vi "Generate Text Coordenates.vi"(8 "Error In":errorcluster, 11 "Pixel In":refnum<class "String.lvclass">) -> (0 "Error Out":errorcluster, 2 "Element To Display":T1[](array[typedef]), 3 "Pixel Out":refnum<class "String.lvclass">)   [LabVIEW 2019, in "String.lvclass"]
uses:
  String.lvclass
  C:/Users/goo13/Documents/GIT Local/myRIO-Neopixel/Source/RT/Display Element/Display Element.lvclass
  Display Utilities/Public/Controls/2D Coordenates.ctl
  Display Utilities/Display Utilities.lvlib
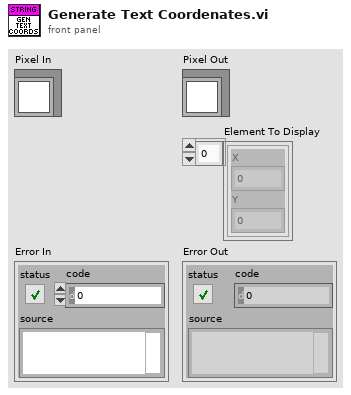
[diagram p1: front panel]
types:
  T1 = typedef "Display Utilities.lvlib/2D Coordenates.ctl" = cluster{"X":i32, "Y":i32}
  T2 = typedef "Display Element.lvclass/Vector.ctl" = cluster{"X":i32, "Y":i32}
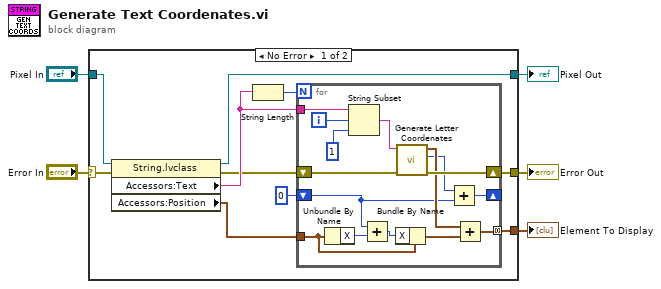
[diagram p0: block diagram]
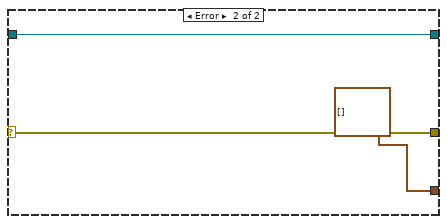
[diagram p2: hidden frame]
diagram:
  n1 = case shown="No Error" "Error In" {
    selector: "Error In" -> [w13 w33]
    tunnel: "Pixel In" -> [w14 w32]
    tunnel: [w7 w33] -> w3
    tunnel: [w15 w32] -> w2
    tunnel: [w8 T1[] []] -> w1
    frame No Error {
      n2 = property class="String.lvclass"(reference=w14, error in=w13) -> (reference out=w15:refnum<class "String.lvclass">, error out=w10:errorcluster, "Accessors:Text"=w11:string, "Accessors:Position"=w9:T2)
      n3 = String Length(string=w11) -> (length=w12:i32)
      n4 = for {
        N: w12 -> [_]
        tunnel: w11 -> [w30]
        shift-right: [w25] -> w7
        shift-left: w10 -> [w26]
        tunnel: w9 -> [w21]
        tunnel: [w23] -> w8 mode=concatenating
        shift-right: [w17] -> _
        shift-left: 0 ("Width") -> [w16]
        i -> [w28]
        n5 = Unbundle By Name(w21) -> ("X"=w22:i32)
        n6 = String Subset(string=w30, offset (0)=w28, length (rest)=1 ("length (rest)")) -> (substring=w27:string)
        n7 = Add(x=w16, y=w22) -> (x+y=w20:i32)
        n8 = Bundle By Name(cluster=w21, "X"=w20) -> (w19:T2)
        n9 = call "Generate Letter Coordenates.vi"("Error In"=w26, "Letter"=w27) -> ("Error Out"=w25:errorcluster, "Width"=w18:i32, "Element To Display"=w24:T1[])  [unwired: 7 in]
        n10 = Add(x=w18, y=w16) -> (x+y=w17:i32)
        n11 = Add(x=w24, y=w19) -> (x+y=w23:T1[])
      }
    }
    frame Error {
    }
  }
  "Pixel Out" <- w2
  "Error Out" <- w3
  "Element To Display" <- w1
